vi "UDP test Half 2.vi"() -> ()   [LabVIEW 2013, in "TEC tests.lvlib"]
uses:
  TEC tests.lvlib
  configuration/TEC configuration.lvclass
  execution/TEC runtime.lvclass
  configuration/TEC configuration.lvclass/TEC configuration.ctl
  <vilib>/NI/Tag Bus/table/data polymorphs/read one/read Double.vi
  configuration/Write receive on port.vi
  configuration/Write send from port.vi
  configuration/Write send to address.vi
  configuration/Write send to port.vi
  <vilib>/NI/Tag Bus/table/data table.lvlib
  <vilib>/ptbypt/NI_PtbyPt.lvlib
  <vilib>/NI/Configuration Framework/serializable configuration/NISE_CEF_serializable configuration.lvclass
panel:
  out "error out 2":errorcluster
  out "error out":errorcluster
  in  "send to address":string="dsmith"
  out "duration avg":dbl
  in  "millisecond multiple":u32=100
  out "duration":dbl
  out "timeout count":u16
  out "final":errorcluster
  out "value rx":dbl
  in  "stop":bool
  out "init err":errorcluster
  in  "ch count":i32=100
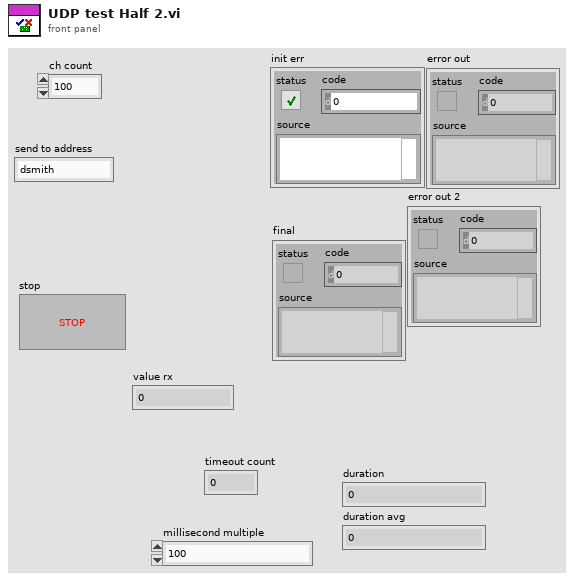
[diagram p1: front panel]
types:
  T1 = typedef "TBM channel.lvclass/data tables.ctl" = cluster{"input data":T2, "processing parameter":T2, "processing result":T2, "output data":T2}
  T2 = typedef "tag bus.lvlib/dictionary table pair.ctl" = cluster{"data dictionary":refnum<class "data dictionary.lvclass">, "data table":T3}
  T3 = typedef "tag bus.lvlib/data table.lvlib/data table.ctl" = cluster{"Double":dbl[], "Single":sgl[], "I64":i64[], "I32":i32[], "I16":i16[], "I8":i8[], "U64":u64[], "U32":u32[], "U16":u16[], "U8":u8[], "Boolean":bool[], "String":string[], "Array of Double":cluster{"DBL Array":dbl[]}[], "Array of Single":cluster{"SGL Array":sgl[]}[], "Array of I64":cluster{"I64 Array":i64[]}[], "Array of I32":cluster{"I32 Array":i32[]}[], "Array of I16":cluster{"I16 Array":i16[]}[], "Array of I8":cluster{"I8 Array":i8[]}[], "Array of U64":cluster{"U64 Array":u64[]}[], "Array of U32":cluster{"U32 Array":u32[]}[], "Array of U16":cluster{"U16 Array":u16[]}[], "Array of U8":cluster{"U8 Array":u8[]}[], "Array of Boolean":cluster{"Boolean Array":bool[]}[], "Array of String":cluster{"String Array":string[]}[]}
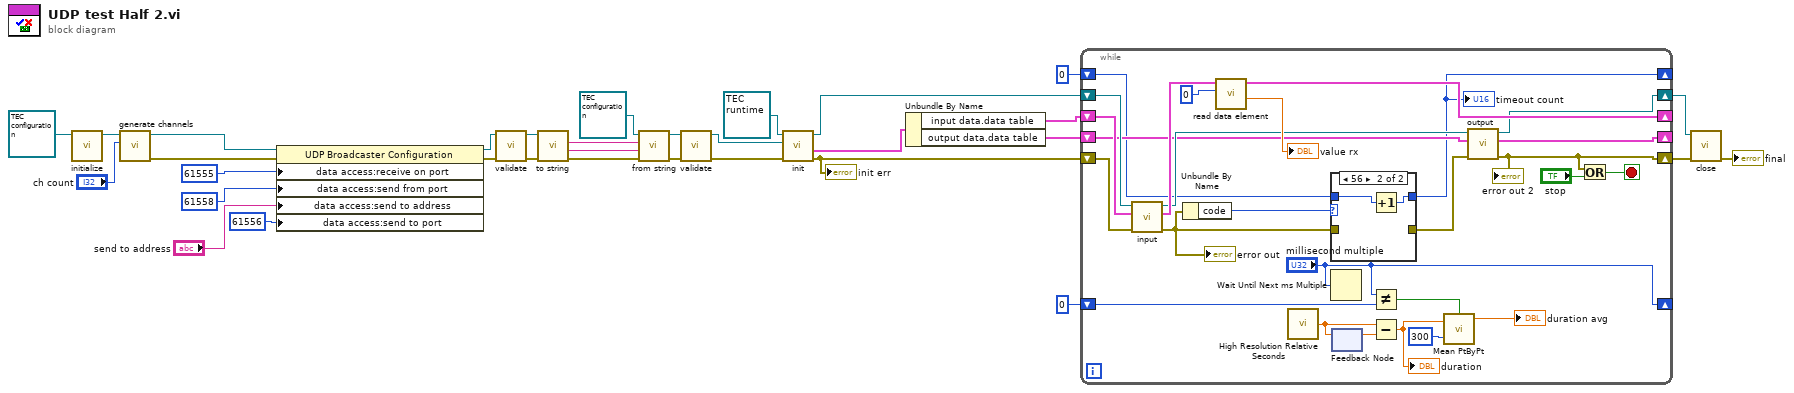
[diagram p0: block diagram]
diagram:
  n1 = call <vilib>:"initialize.vi"("configuration in"=refnum<class "TEC configuration.lvclass"> refnum ("tag bus configurable plugin module configuration")) -> ("configuration out"=w2:refnum<class "TEC configuration.lvclass">)  [unwired: 8 in, 2 out]
  n2 = call "generate channels.vi"("ch count"="ch count", "TEC configuration in"=w2) -> ("error out"=w4:errorcluster, "TEC configuration out"=w3:refnum<class "TEC configuration.lvclass">)  [unwired: 8 in]
  n3 = property class="UDP Broadcaster Configuration"(reference=w3, error in=w4, "data access:receive on port"=u16 61555 ("send from port"), "data access:send from port"=u16 61558 ("send to port"), "data access:send to address"="send to address", "data access:send to port"=u16 61556 ("receive on port")) -> (reference out=w20:refnum<class "TEC configuration.lvclass">, error out=w21:errorcluster)
  n4 = call-dynamic "validate.vi"("error in"=w21, "TEC configuration in"=w20) -> ("error out"=w22:errorcluster, "TEC configuration out"=w28:refnum<class "TEC configuration.lvclass">)  [unwired: 8 in]
  n5 = call-dynamic "to string.vi"("error in"=w22, "TEC configuration in"=w28) -> ("error out"=w25:errorcluster, "data"=w24:string, "version"=w23:string)  [unwired: 6 in, 1 out]
  n6 = call-dynamic "from string.vi"("error in"=w25, "data"=w24, "version"=w23, "TEC configuration in"=refnum<class "TEC configuration.lvclass"> refnum) -> ("error out"=w27:errorcluster, "TEC configuration out"=w26:refnum<class "TEC configuration.lvclass">)  [unwired: 6 in]
  n7 = call-dynamic "validate.vi"("error in"=w27, "TEC configuration in"=w26) -> ("error out"=w18:errorcluster, "TEC configuration out"=w17:refnum<class "TEC configuration.lvclass">)  [unwired: 8 in]
  n8 = call-dynamic "init.vi"("error in"=w18, "TBM module configuration in"=w17, "TEC runtime in"=refnum<class "TEC runtime.lvclass"> refnum ("tag bus configurable plugin module")) -> ("error out"=w16:errorcluster, "data allocations"=w14:T1, "TEC runtime out"=w11:refnum<class "TEC runtime.lvclass">)  [unwired: 5 in, 1 out]
  "init err" <- w16
  n9 = Unbundle By Name(w14) -> ("input data.data table"=w13:T3, "output data.data table"=w12:T3)
  n10 = while {
    shift-right: [w57] -> _
    shift-left: w13 -> [w53]
    shift-right: [w49] -> _
    shift-left: w12 -> [w47]
    shift-right: [w50] -> w8
    shift-left: w11 -> [w55]
    shift-right: [w48] -> w10
    shift-left: w16 -> [w54]
    shift-right: [w43] -> _
    shift-left: u16 0 ("Numeric") -> [w42]
    shift-right: ["millisecond multiple"] -> _
    shift-left: u32 0 ("millisecond multiple") -> [w36]
    stop <- w58 stop-if-true
    n11 = call-dynamic "input.vi"("error in"=w54, "data table in"=w53, "TEC runtime in"=w55) -> ("error out"=w45:errorcluster, "data table out"=w52:T3, "TEC runtime out"=w51:refnum<class "TEC runtime.lvclass">)  [unwired: 6 in]
    "error out" <- w45
    n12 = Unbundle By Name(w45) -> ("code"=w46:i32)
    n13 = call-poly <vilib>:"read data element.vi"("index"=0, "data table in"=w52) -> ("value"=→"value rx":dbl, "data table out"=w57:T3)  [unwired: 8 in]
    n14 = call <vilib>:"High Resolution Relative Seconds.vi"() -> ("relative seconds"=w40:dbl)
    n15 = case shown="56" w46 {
      tunnel: w45 -> [w61 _]
      tunnel: [w61 _] -> w44
      tunnel: [w60 w63] -> w43
      tunnel: w42 -> [w60 w62]
      frame 0, Default {
      }
      frame 56 {
        n16 = Increment(x=w62) -> (x+1=w63:u16)
      }
    }
    "timeout count" <- w43
    n17 = Wait Until Next ms Multiple(millisecond multiple="millisecond multiple") -> ()  [unwired: 1 out]
    n18 = feedback-in #1(w40) -> ()
    n19 = feedback #1() -> (w41:dbl)  [unwired: 1 in]
    n20 = Not Equal?(x="millisecond multiple", y=w36) -> (x != y?=w35:bool)
    n21 = Subtract(x=w40, y=w41) -> (x-y=w39:dbl)
    "duration" <- w39
    n22 = call <vilib>:"Mean PtByPt.vi"("x"=w39, "sample length"=300, "initialize"=w35) -> ("mean"=→"duration avg":dbl)  [unwired: 1 in, 1 out]
    n23 = call-dynamic "output.vi"("error in"=w44, "data table in"=w47, "TEC runtime in"=w51) -> ("error out"=w48:errorcluster, "data table out"=w49:T3, "TEC runtime out"=w50:refnum<class "TEC runtime.lvclass">)  [unwired: 6 in]
    "error out 2" <- w48
    n24 = Or(x=w48, y="stop") -> (x .or. y?=w58:bool)
  }
  n25 = call-dynamic "close.vi"("error in"=w10, "TEC runtime in"=w8) -> ("error out"=→"final":errorcluster)  [unwired: 9 in]
